vi "DVR Flatten.vi"(7 "payload in":u8[](array[numeric]), 8 "error in (no error)":errorcluster, 10 "Data In":refnum<data-value>[](array[refnum]), 11 "CIFFifo in":refnum<class "CIFfifo.lvclass">) -> (0 "error out":errorcluster, 1 "Total Length":i32, 2 "Data Out":refnum<data-value>[](array[refnum]), 3 "CIFFifo out":refnum<class "CIFfifo.lvclass">, 5 "payload out":u8[](array[numeric]))   [LabVIEW 2021, in "CIFfifo.lvclass"]
uses:
  CIFfifo.lvclass
  typedef/Datatype Waveform.ctl
  CIFfifo.lvclass/CIFfifo.ctl
  6fdbece9-bad6-4a8e-9bf7-fe1528478dd6.vi
  Accessors/Write Payload Length.vi
  Accessors/Read Header.vi
  CIFCore/Common/Utilities/Add Error.vi
  6fdbece9-bad6-4a8e-9bf7-fe1528478dd6.vi/c28b0ead-42ad-4072-80a2-aca7f2bd7ce3.vi
  CIFCore/Common/Utilities/Append Error Location.vi
  ChannelCommon.lvlib
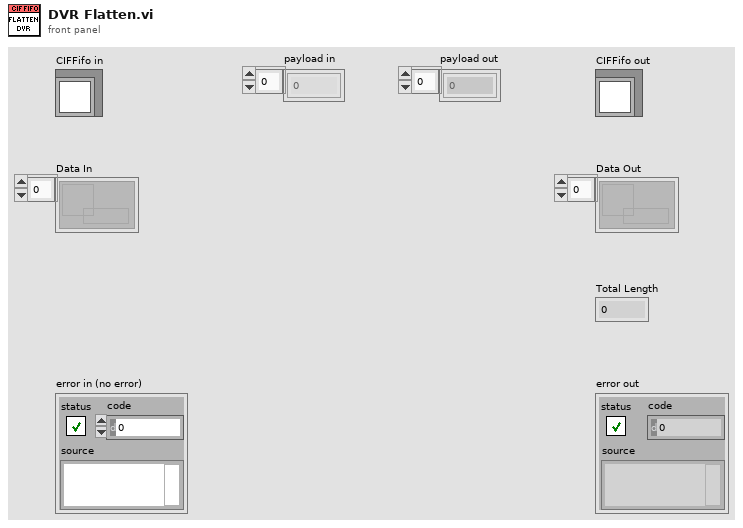
[diagram p1: front panel]
types:
  T1 = typedef "ChannelCommon.lvlib/FIFO Header.ctl" = cluster{"Length":u64, "T0":u64, "T_Out":u64, "T_Tx":u64, "Ctr":u64, "ClockID":u8}
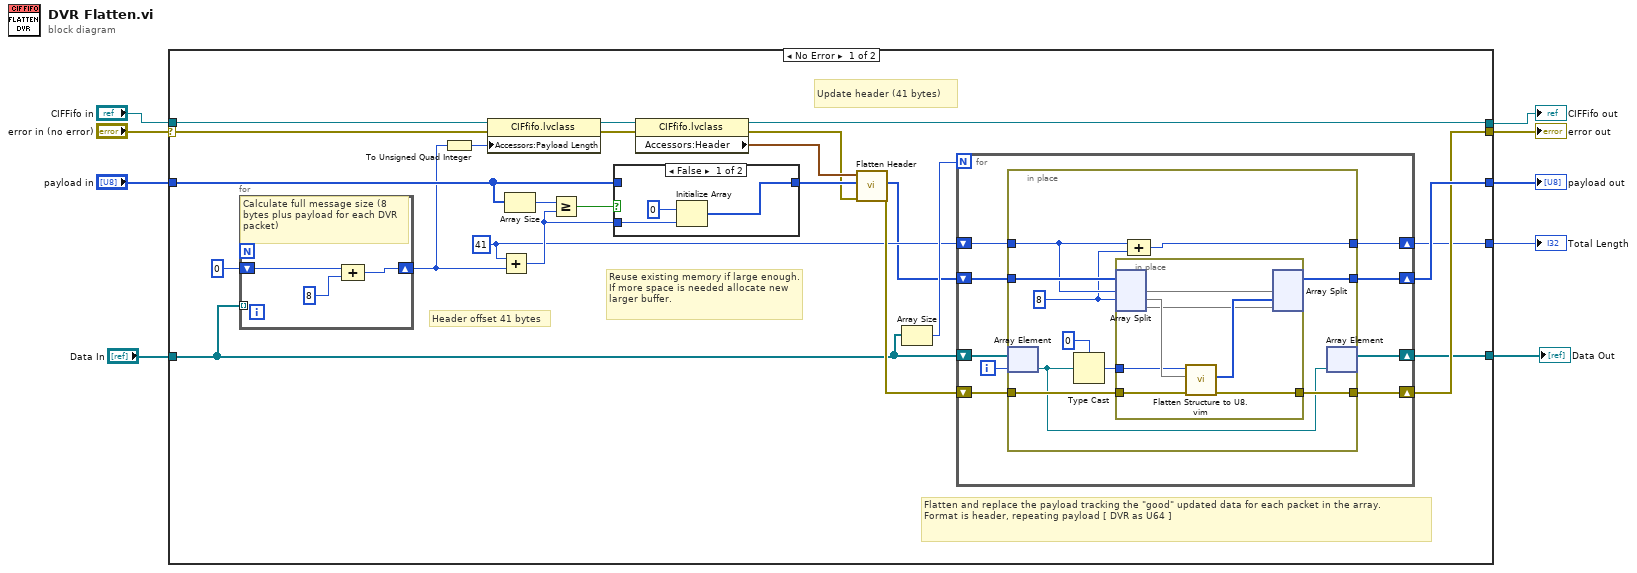
[diagram p0: block diagram]
diagram:
  n1 = case shown="No Error" "error in (no error)" {
    selector: "error in (no error)" -> [w24 w70]
    tunnel: [w17 w70] -> w8
    tunnel: "Data In" -> [w10 w67]
    tunnel: "CIFFifo in" -> [w33 w69]
    tunnel: [w21 w69] -> w4
    tunnel: [w18 w68] -> w6
    tunnel: "payload in" -> [w25 w68]
    tunnel: [w16 w67] -> w1
    tunnel: [w13 _] -> w3
    frame No Error {
      w15 = 41 ("y")
      # "Flatten and replace the payload tracking the \"good\" updated data for each packet in the array.\nFormat is header, repeating payload [ DVR as U64 ]"
      # "Header offset 41 bytes"
      # "Update header (41 bytes)"
      # "Reuse existing memory if large enough.  If more space is needed allocate new larger buffer."
      n2 = for {
        tunnel: w10 -> [_] mode=indexing
        shift-right: [w36] -> w11
        shift-left: 0 -> [w35]
        # "Calculate full message size (8 bytes plus payload for each DVR packet)"
        n3 = Compound Arithmetic op=ADD(w35, 8 ("value")) -> (w36:i32)
      }
      n4 = To Unsigned Quad Integer(1:w11) -> (0:w31:u64)
      n5 = property class="CIFfifo.lvclass"(reference=w33, error in=w24, "Accessors:Payload Length"=w31) -> (reference out=w23:refnum<class "CIFfifo.lvclass">, error out=w22:errorcluster)
      n6 = Add(x=w15, y=w11) -> (x+y=w26:i32)
      n7 = Array Size(array=w25) -> (size(s)=w30:i32)
      n8 = Greater Or Equal?(x=w30, y=w26) -> (x >= y?=w29:bool)
      n9 = case shown="False" w29 {
        tunnel: w25 -> [_ w66]
        tunnel: [w63 w66] -> w28
        tunnel: w26 -> [w65 _]
        frame False {
          n10 = Initialize Array(u8 0, w65) -> (w63:u8[])
        }
        frame True {
        }
      }
      n11 = property class="CIFfifo.lvclass"(reference=w23, error in=w22) -> (reference out=w21:refnum<class "CIFfifo.lvclass">, error out=w27:errorcluster, "Accessors:Header"=w32:T1)
      n12 = call "Flatten Header.vi"("error in"=w27, "Flattened Data in"=w28, "Header in"=w32) -> ("error out"=w19:errorcluster, "Flattened Data out"=w14:u8[])  [unwired: 6 in, 1 out]
      n13 = Array Size(array=w10) -> (size(s)=w20:i32)
      n14 = for {
        N: w20 -> [_]
        shift-right: [w45] -> w17
        shift-left: w19 -> [w44]
        shift-right: [w42] -> w18
        shift-left: w14 -> [w43]
        shift-right: [w40] -> w13
        shift-left: w15 -> [w41]
        shift-right: [w37] -> w16
        shift-left: w10 -> [w39]
        i -> [w38]
        n15 = in-place {
          in-place-border: [w55] -> w45
          in-place-border: w44 -> [w54]
          in-place-border: w43 -> [w53]
          in-place-border: [w52] -> w42
          in-place-border: w41 -> [w51]
          in-place-border: [w50] -> w40
          w49 = 8 ("value")
          n16 = in-place-array #1(w39, w38) -> (w46:refnum<data-value>)
          n17 = Type Cast(type=u64 0, x=w46) -> (*(type *) &x=w47:u64)
          n18 = in-place {
            in-place-border: w54 -> [w61]
            in-place-border: [w58] -> w55
            in-place-border: w47 -> [w56]
            n19 = in-place-split #2(w53, w51, w49) -> (w62:u8[], w59:u8[], w57:u8[])
            n20 = call "Flatten Structure to U8.vim"("error in"=w61, "Flattened Data in"=w59, "Data to Flatten in"=w56) -> ("error out"=w58:errorcluster, "Flattened Data out"=w60:u8[])  [unwired: 6 in, 1 out]
            n21 = in-place-split #2(w62, w60, w57) -> (w52:u8[])  [unwired: 2 out]
          }
          n22 = Compound Arithmetic op=ADD(w51, w49) -> (w50:i32)
          n23 = in-place-array #1(w46) -> (w37:refnum<data-value>[])  [unwired: 1 out]
        }
      }
    }
    frame Error {
    }
  }
  "error out" <- w8
  "CIFFifo out" <- w4
  "payload out" <- w6
  "Total Length" <- w3
  "Data Out" <- w1
